vi "myRIO_BRig_RT__Case_Exp_State_initTrial_LC_Cue1_2.vi"(0 "input_CueType_Switch":u16, 1 "input_Probability_Switch":u16, 2 "input_Count_Switch":u16, 3 "input_CueType_NS":u16, 4 "input_Probability_NS":u16, 5 "input_Count_NS":u16, 6 "input_spout":enum16{"Left", "Right"}(ring), 7 "input_dataBlock":u16[][](array[numeric]), 8 "input_dataCurrent":u16[](array[numeric]), 9 "input_arrTrig":bool[](array[boolean])) -> (10 "output_dataCurrent":u16[](array[numeric]), 11 "output_arrTrig":bool[](array[boolean]))   [LabVIEW 2014]
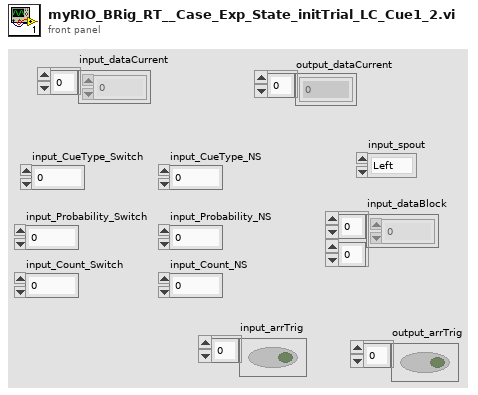
[diagram p1: front panel]
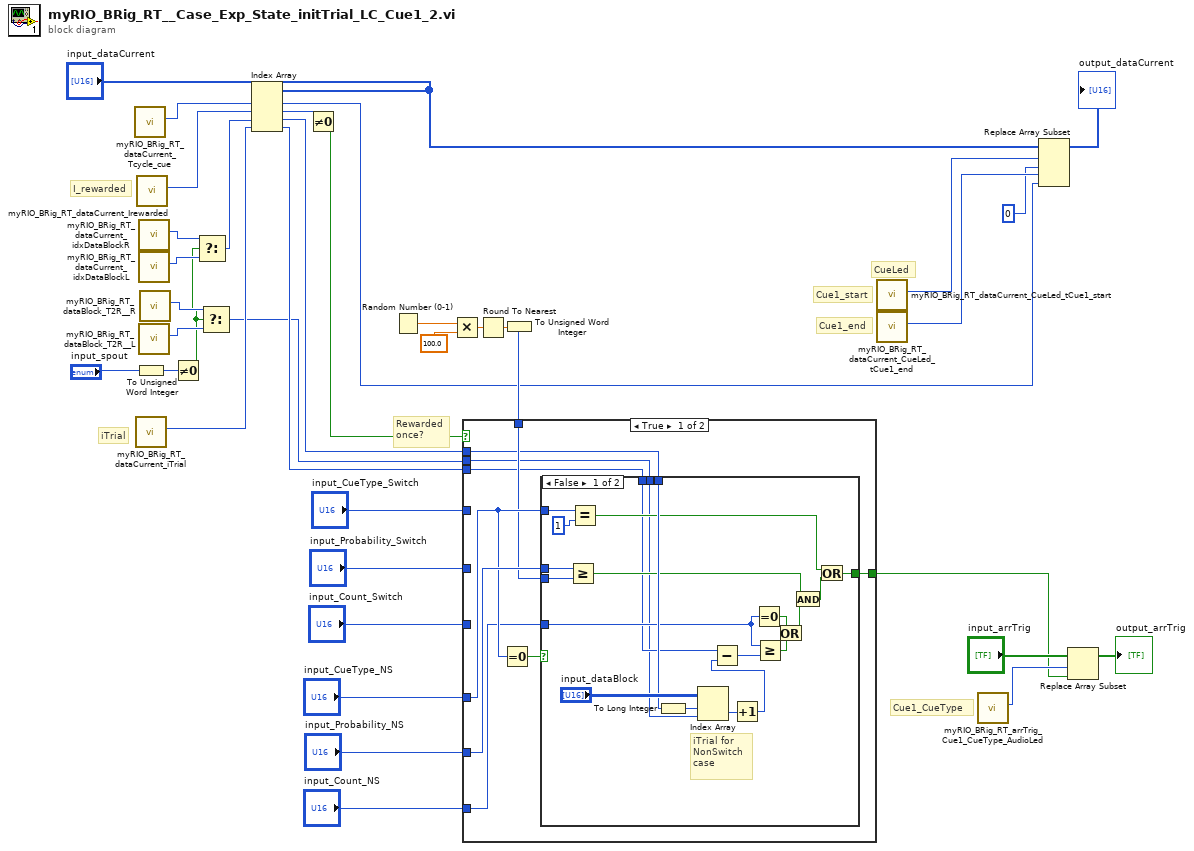
[diagram p0: block diagram]
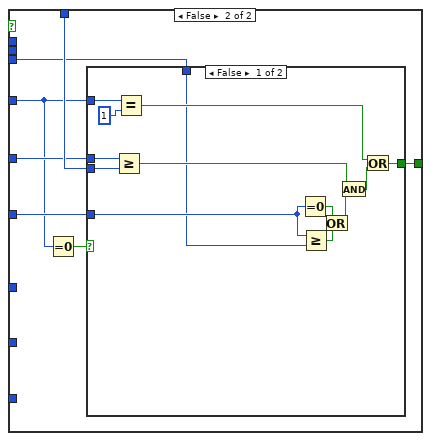
[diagram p3: hidden frame]
diagram:
  # "iTrial"
  # "Cue1_end"
  # "Cue1_start"
  # "CueLed"
  # "Cue1_CueType"
  # "Rewarded\nonce?"
  # "I_rewarded"
  n1 = call "myRIO_BRig_RT_dataCurrent_Tcycle_cue.vi"() -> ("output_Tcycle_cue"=w1:i32)  [unwired: 11 in]
  n2 = To Unsigned Word Integer(number="input_spout") -> (unsigned 16bit integer=w10:u16)
  n3 = call "myRIO_BRig_RT_dataCurrent_iTrial.vi"() -> ("output_iTrial"=w4:i32)  [unwired: 11 in]
  n4 = call "myRIO_BRig_RT_dataCurrent_Irewarded.vi"() -> ("output_I_rewarded"=w15:i32)  [unwired: 11 in]
  n5 = call "myRIO_BRig_RT_dataCurrent_idxDataBlockR.vi"() -> ("output_idxDataBlock__R"=w8:i32)  [unwired: 11 in]
  n6 = call "myRIO_BRig_RT_dataCurrent_idxDataBlockL.vi"() -> ("output_idxDataBlock__L"=w7:i32)  [unwired: 11 in]
  n7 = call "myRIO_BRig_RT_dataBlock_T2R__L.vi"() -> ("output_T2R__L"=w11:i32)  [unwired: 11 in]
  n8 = call "myRIO_BRig_RT_dataBlock_T2R__R.vi"() -> ("output_T2R__R"=w9:i32)  [unwired: 11 in]
  n9 = Not Equal To 0?(x=w10) -> (x != 0?=w6:bool)
  n10 = Select(t=w8, s=w6, f=w7) -> (s? t:f=w5:i32)
  n11 = Select(t=w9, s=w6, f=w11) -> (s? t:f=w2:i32)
  n12 = Index Array(array="input_dataCurrent", index #1=w1, index #2=w15, index #3=w5, index #4=w4) -> (element #1=w17:u16, element #2=w14:u16, element #3=w13:u16, element #4=w3:u16)
  n13 = Not Equal To 0?(x=w14) -> (x != 0?=w33:bool)
  n14 = Random Number (0-1)() -> (number: 0 to 1=w29:dbl)
  n15 = Multiply(x=w29, y=100.0) -> (x*y=w30:dbl)
  n16 = Round To Nearest(number=w30) -> (nearest integer value=w31:dbl)
  n17 = To Unsigned Word Integer(number=w31) -> (unsigned 16bit integer=w28:u16)
  n18 = case shown="True" w33 {
    tunnel: w28 -> [w42 w71]
    tunnel: "input_CueType_Switch" -> [_ w67]
    tunnel: "input_Probability_Switch" -> [_ w68]
    tunnel: "input_Count_Switch" -> [_ w69]
    tunnel: "input_CueType_NS" -> [w43 _]
    tunnel: "input_Probability_NS" -> [w44 _]
    tunnel: "input_Count_NS" -> [w41 _]
    tunnel: [w45 w72] -> w18
    tunnel: w13 -> [w40 _]
    tunnel: w2 -> [w39 _]
    tunnel: w3 -> [w38 w70]
    frame True {
      n19 = Equal To 0?(x=w43) -> (x = 0?=w46:bool)
      n20 = case shown="False" w46 {
        tunnel: w43 -> [w66 _]
        tunnel: w44 -> [w63 _]
        tunnel: [w53 _] -> w45
        tunnel: w42 -> [w64 _]
        tunnel: w41 -> [w58 _]
        tunnel: w40 -> [w59 _]
        tunnel: w39 -> [w47 _]
        tunnel: w38 -> [w50 _]
        frame False {
          # "iTrial for\nNonSwitch\ncase"
          n21 = Greater Or Equal?(x=w63, y=w64) -> (x >= y?=w54:bool)
          n22 = Equal?(x=w66, y=u16 1) -> (x = y?=w51:bool)
          n23 = To Long Integer(number=w59) -> (32bit integer=w62:i32)
          n24 = Index Array(array="input_dataBlock", index (row)=w62, index (col)=w47) -> (element=w61:u16)
          n25 = Increment(x=w61) -> (x+1=w49:u16)
          n26 = Subtract(x=w50, y=w49) -> (x-y=w48:u16)
          n27 = Equal To 0?(x=w58) -> (x = 0?=w56:bool)
          n28 = Greater Or Equal?(x=w58, y=w48) -> (x >= y?=w57:bool)
          n29 = Or(x=w56, y=w57) -> (x .or. y?=w55:bool)
          n30 = And(x=w54, y=w55) -> (x .and. y?=w52:bool)
          n31 = Or(x=w51, y=w52) -> (x .or. y?=w53:bool)
        }
        frame True {
        }
      }
    }
    frame False {
      n32 = Equal To 0?(x=w67) -> (x = 0?=w73:bool)
      n33 = case shown="False" w73 {
        tunnel: w67 -> [w86 _]
        tunnel: w68 -> [w83 _]
        tunnel: [w77 _] -> w72
        tunnel: w71 -> [w84 _]
        tunnel: w69 -> [w82 _]
        tunnel: w70 -> [w74 _]
        frame False {
          n34 = Greater Or Equal?(x=w83, y=w84) -> (x >= y?=w78:bool)
          n35 = Equal?(x=w86, y=u16 1) -> (x = y?=w75:bool)
          n36 = Equal To 0?(x=w82) -> (x = 0?=w80:bool)
          n37 = Greater Or Equal?(x=w82, y=w74) -> (x >= y?=w81:bool)
          n38 = Or(x=w80, y=w81) -> (x .or. y?=w79:bool)
          n39 = And(x=w78, y=w79) -> (x .and. y?=w76:bool)
          n40 = Or(x=w75, y=w76) -> (x .or. y?=w77:bool)
        }
        frame True {
        }
      }
    }
  }
  n41 = call "myRIO_BRig_RT_dataCurrent_CueLed_tCue1_start.vi"() -> ("output_CueLed_tCue1_start"=w27:i32)  [unwired: 11 in]
  n42 = call "myRIO_BRig_RT_dataCurrent_CueLed_tCue1_end.vi"() -> ("output_CueLed_tCue1_end"=w26:i32)  [unwired: 11 in]
  n43 = call "myRIO_BRig_RT_arrTrig_Cue1_CueType_AudioLed.vi"() -> ("output_arrTrig_Cue1_CueType_AudioLed"=w25:i32)  [unwired: 11 in]
  n44 = Replace Array Subset(array="input_dataCurrent", new element #1=u16 0 ("new element/subarray"), index #1=w27, new element #2=w17, index #2=w26) -> (→"output_dataCurrent":u16[])
  n45 = Replace Array Subset(array="input_arrTrig", new element=w18, index=w25) -> (→"output_arrTrig":bool[])
